vi "Main_Module.vi"(0 "File_Path":path caption="File Path", 1 "Moving_Average":i32=10 caption="Moving Average" min=5 max=500, 5 "Input_Size (in kb)":i64=100 caption="Input Size (in kb)" min=10 max=1048576, 7 "Upper_Limit":dbl=100.0 caption="Upper Limit" min=1.0 max=100.0, 9 "Lower_Limit":dbl caption="Lower Limit" min=0.0 max=99.0, 11 "Error_In":errorcluster, 12 "Stop":bool) -> (4 "Generated_Data":dbl[](graph) caption="Generated Data", 15 "Error_Out":errorcluster)   [LabVIEW 2021]
doc: "This is the main vi that user can interact."
uses:
  Controls/Operation_Select_Queue.ctl
  Controls/Operation_Select_Stack.ctl
panel:
  out "Generated_Number":dbl caption="Generated Number"
  # "ADQ System"
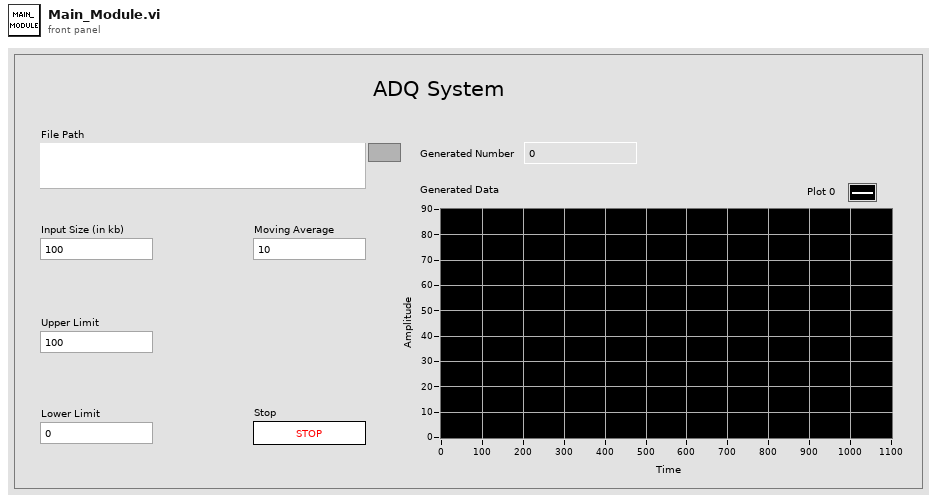
[diagram p1: front panel]
types:
  T1 = typedef "Operation_Select_Stack.ctl" = enum16{"Initialize", "Push", "Pop", "Preview"}
  T2 = typedef "Operation_Select_Queue.ctl" = enum16{"Initialize", "Enqueue", "Dequeue", "Preview"}
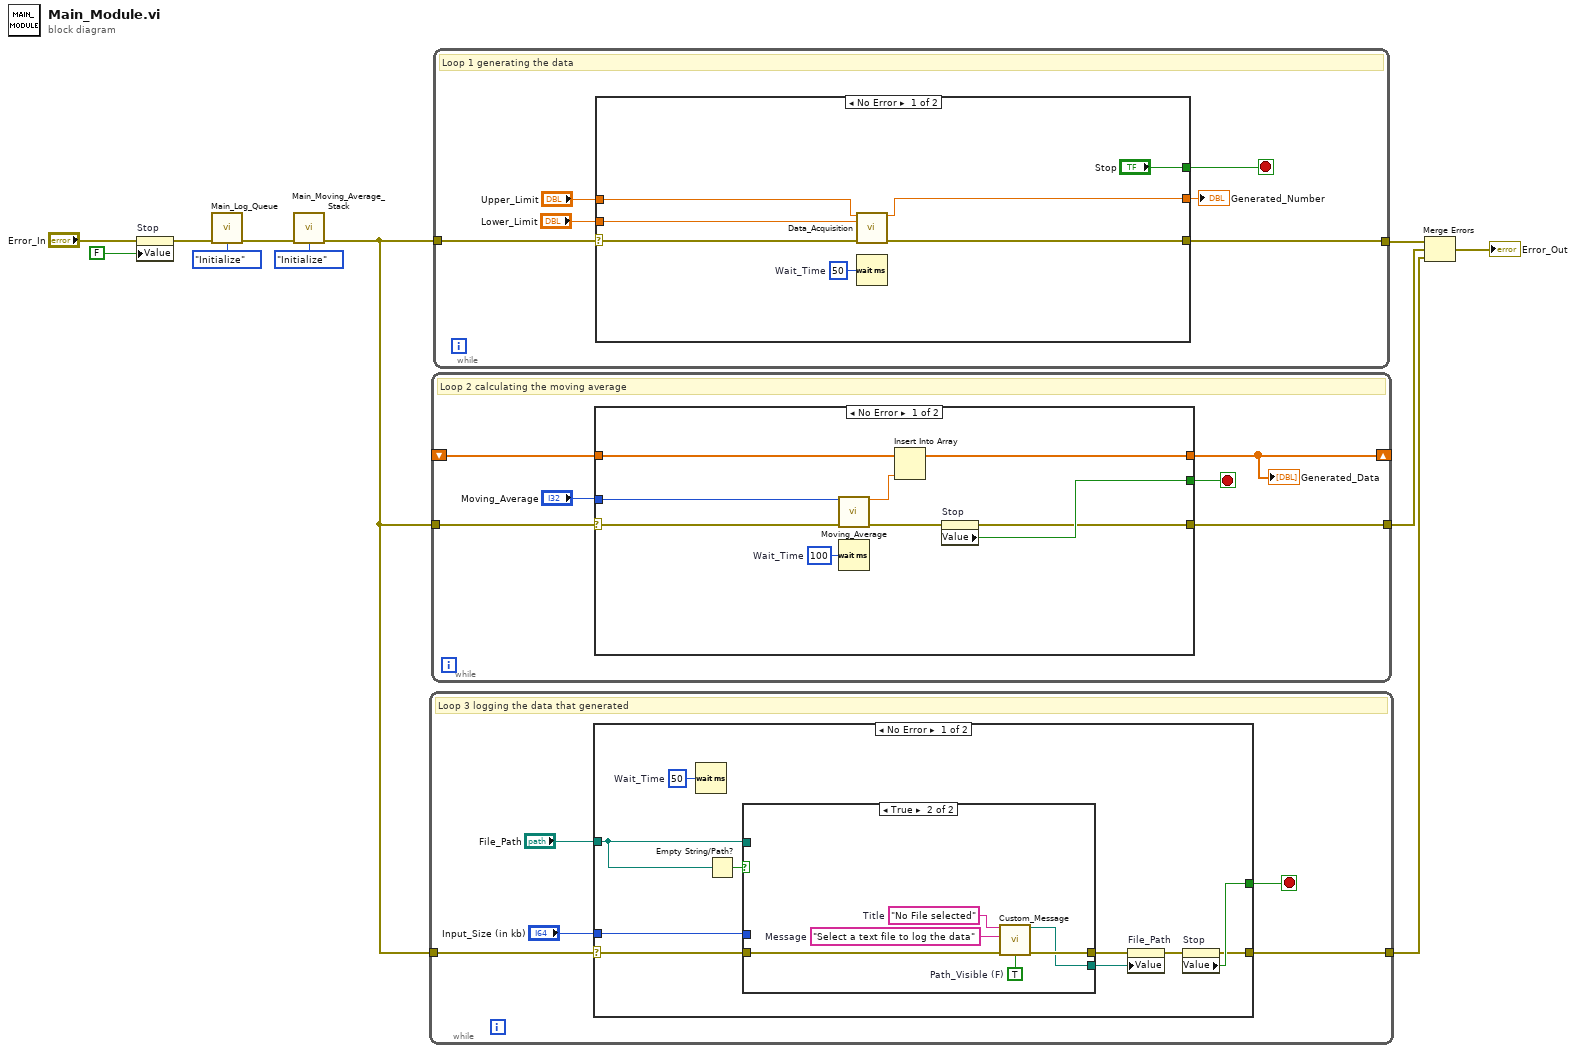
[diagram p0: block diagram]
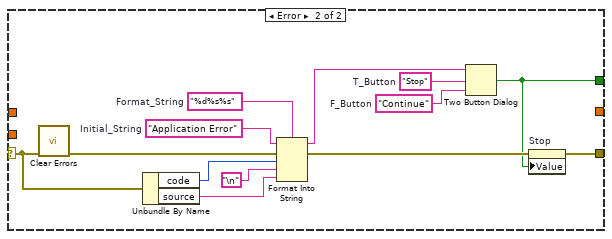
[diagram p2: hidden frame]
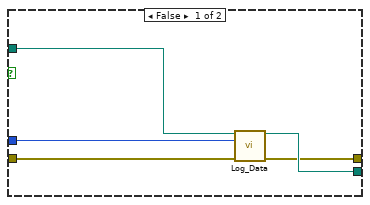
[diagram p3: hidden frame]
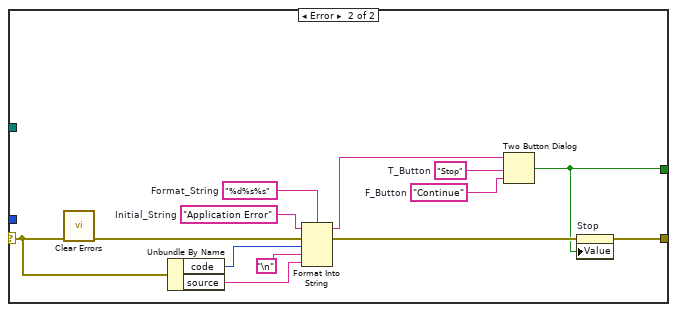
[diagram p4: hidden frame]
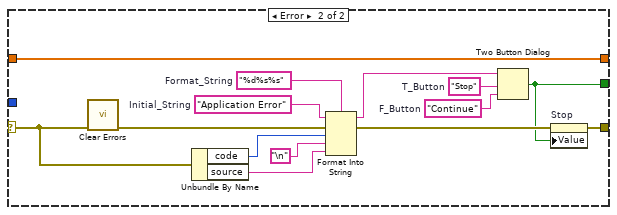
[diagram p5: hidden frame]
diagram:
  n1 = property on="Stop" class="Bool (strict)"(error in="Error_In", "Value"=FALSE ("Stop")) -> (error out=w6:errorcluster)  [unwired: 1 in, 1 out]
  n2 = call "Main_Log_Queue.vi"("Error_In"=w6, "Operation"=Operation_Select_Queue."Initialize") -> ("Error_Out"=w10:errorcluster)  [unwired: 9 in, 4 out]
  n3 = call "Main_Moving_Average_Stack.vi"("Error_In"=w10, "Operation"=Operation_Select_Stack."Initialize") -> ("Error_Out"=w4:errorcluster)  [unwired: 9 in, 4 out]
  n4 = while {
    tunnel: w4 -> [w16]
    tunnel: [w15] -> w1
    stop <- w14 stop-if-true
    # "Loop 3 logging the data that generated"
    n5 = case shown="No Error" w16 {
      selector: w16 -> [w26 w38]
      tunnel: [w22 w40] -> w15
      tunnel: [w23 w39] -> w14
      tunnel: "Input_Size (in kb)" -> [w18 _]
      tunnel: "File_Path" -> [w17 _]
      frame No Error {
        w24 = u32 50  # Wait_Time
        n6 = Wait (ms)(milliseconds to wait=w24) -> ()  [unwired: 1 out]
        n7 = Empty String/Path?(string/path=w17) -> (empty?=w25:bool)
        n8 = case shown="True" w25 {
          tunnel: w26 -> [w31 w34]
          tunnel: w17 -> [w30 _]
          tunnel: w18 -> [w29 _]
          tunnel: [w27 w37] -> w19
          tunnel: [w28 w32] -> w21
          frame False {
            n9 = call "Log_Data.vi"("File_Path_In"=w30, "Input_Size (in kb)"=w29, "Error_In"=w31) -> ("File_Path_Out"=w28:path, "Error_Out"=w27:errorcluster)  [unwired: 11 in]
          }
          frame True {
            w33 = TRUE  # Path_Visible (F)
            w35 = "Select a text file to log the data"  # Message
            w36 = "No File selected"  # Title
            n10 = call "Custom_Message.vi"("Title"=w36, "Message"=w35, "Error_In"=w34, "Path_Visible (F)"=w33) -> ("Path_Out"=w32:path, "Error_Out"=w37:errorcluster)  [unwired: 10 in]
          }
        }
        n11 = property on="File_Path" class="Path"(error in=w19, "Value"=w21) -> (error out=w20:errorcluster)  [unwired: 1 in, 1 out]
        n12 = property on="Stop" class="Bool (strict)"(error in=w20) -> (error out=w22:errorcluster, "Value"=w23:bool)  [unwired: 1 in, 1 out]
      }
      frame Error {
        w46 = "%d%s%s"  # Format_String
        w47 = "Application Error"  # Initial_String
        w48 = "Stop"  # T_Button
        w49 = "Continue"  # F_Button
        n13 = call <vilib>:"Clear Errors.vi"("error in (no error)"=w38) -> ("error out"=w44:errorcluster)  [unwired: 5 in, 1 out]
        n14 = Unbundle By Name(w38) -> ("code"=w43:i32, "source"=w42:string)
        n15 = Format Into String(format string=w46, initial string=w47, error in=w44, w43, "\n", w42) -> (resulting string=w50:string, error out=w41:errorcluster)
        n16 = Two Button Dialog(message=w50, 1:w49, 2:w48) -> (T button?=w39:bool)
        n17 = property on="Stop" class="Bool (strict)"(error in=w41, "Value"=w39) -> (error out=w40:errorcluster)  [unwired: 1 in, 1 out]
      }
    }
  }
  n18 = while {
    tunnel: w4 -> [w56]
    tunnel: [w55] -> w2
    shift-right: [w52] -> _
    shift-left: _ -> [w54]
    stop <- w53 stop-if-true
    # "Loop 2 calculating the moving average"
    n19 = case shown="No Error" w56 {
      selector: w56 -> [w65 w67]
      tunnel: [w58 w68] -> w55
      tunnel: [w62 w79] -> w52
      tunnel: w54 -> [w64 w79]
      tunnel: [w60 w66] -> w53
      tunnel: "Moving_Average" -> [w57 _]
      frame No Error {
        w61 = u32 100  # Wait_Time
        n20 = call "Moving_Average.vi"("Moving_Average"=w57, "Error_In"=w65) -> ("Moving_Average_Value"=w63:dbl, "Error_Out"=w59:errorcluster)  [unwired: 12 in]
        n21 = Wait (ms)(milliseconds to wait=w61) -> ()  [unwired: 1 out]
        n22 = Insert Into Array(array=w64, new element=w63) -> (w62:dbl[])  [unwired: 1 in]
        n23 = property on="Stop" class="Bool (strict)"(error in=w59) -> (error out=w58:errorcluster, "Value"=w60:bool)  [unwired: 1 in, 1 out]
      }
      frame Error {
        w74 = "%d%s%s"  # Format_String
        w75 = "Application Error"  # Initial_String
        w76 = "Stop"  # T_Button
        w77 = "Continue"  # F_Button
        n24 = call <vilib>:"Clear Errors.vi"("error in (no error)"=w67) -> ("error out"=w72:errorcluster)  [unwired: 5 in, 1 out]
        n25 = Unbundle By Name(w67) -> ("code"=w71:i32, "source"=w70:string)
        n26 = Format Into String(format string=w74, initial string=w75, error in=w72, w71, "\n", w70) -> (resulting string=w78:string, error out=w69:errorcluster)
        n27 = Two Button Dialog(message=w78, 1:w77, 2:w76) -> (T button?=w66:bool)
        n28 = property on="Stop" class="Bool (strict)"(error in=w69, "Value"=w66) -> (error out=w68:errorcluster)  [unwired: 1 in, 1 out]
      }
    }
    "Generated_Data" <- w52
  }
  n29 = while {
    tunnel: w4 -> [w85]
    tunnel: [w84] -> w3
    stop <- w83 stop-if-true
    # "Loop 1 generating the data"
    n30 = case shown="No Error" w85 {
      selector: w85 -> [w92 w93]
      tunnel: [w91 w95] -> w84
      tunnel: ["Stop" w94] -> w83
      tunnel: "Lower_Limit" -> [w88 _]
      tunnel: "Upper_Limit" -> [w87 _]
      tunnel: [w86 _] -> w80
      frame No Error {
        w90 = u32 50  # Wait_Time
        n31 = call "Data_Acquisition.vi"("Upper_Limit"=w87, "Lower_Bound"=w88, "Error_In"=w92) -> ("Generated_Number"=w86:dbl, "Error_Out"=w91:errorcluster)  [unwired: 11 in]
        n32 = Wait (ms)(milliseconds to wait=w90) -> ()  [unwired: 1 out]
      }
      frame Error {
        w101 = "%d%s%s"  # Format_String
        w102 = "Application Error"  # Initial_String
        w103 = "Stop"  # T_Button
        w104 = "Continue"  # F_Button
        n33 = call <vilib>:"Clear Errors.vi"("error in (no error)"=w93) -> ("error out"=w99:errorcluster)  [unwired: 5 in, 1 out]
        n34 = Unbundle By Name(w93) -> ("code"=w98:i32, "source"=w97:string)
        n35 = Format Into String(format string=w101, initial string=w102, error in=w99, w98, "\n", w97) -> (resulting string=w105:string, error out=w96:errorcluster)
        n36 = Two Button Dialog(message=w105, 1:w104, 2:w103) -> (T button?=w94:bool)
        n37 = property on="Stop" class="Bool (strict)"(error in=w96, "Value"=w94) -> (error out=w95:errorcluster)  [unwired: 1 in, 1 out]
      }
    }
    "Generated_Number" <- w80
  }
  n38 = Merge Errors(w3, w2, w1) -> (→"Error_Out":errorcluster)
